vi "Plot Style Chooser Dialog.vi"(3 "Error In":errorcluster) -> (6 "Plot Style out":T1={"Plot Style"=enum."unchanged", "Histogram Type"=enum."Left Bound", "Line Tickness"=enum."unchanged", "Line Style"=enum."unchanged", "Point Style"=enum."unchanged", "Line Color"=0, "Point Color"=0, "Anti-aliased"=FALSE, "Line Color Chooser"=enum."unchanged", "Point Color Chooser"=enum."unchanged", "Line Color List"="", "Point Color List"=""}, 7 "Cancelled?":bool, 9 "Error Out":errorcluster)   [LabVIEW 2019]
uses:
  Plot Style 3.ctl
  <vilib>/measure/NI_MABase.lvlib
panel:
  in  "Cancel":bool
  in  "OK":bool
  out "Preview":waveform(dbl)(graph)
  in  "Plot Style":T1={"Plot Style"=enum."unchanged", "Histogram Type"=enum."Left Bound", "Line Tickness"=enum."unchanged", "Line Style"=enum."unchanged", "Point Style"=enum."unchanged", "Line Color"=0, "Point Color"=0, "Anti-aliased"=FALSE, "Line Color Chooser"=enum."unchanged", "Point Color Chooser"=enum."unchanged", "Line Color List"="", "Point Color List"=""}
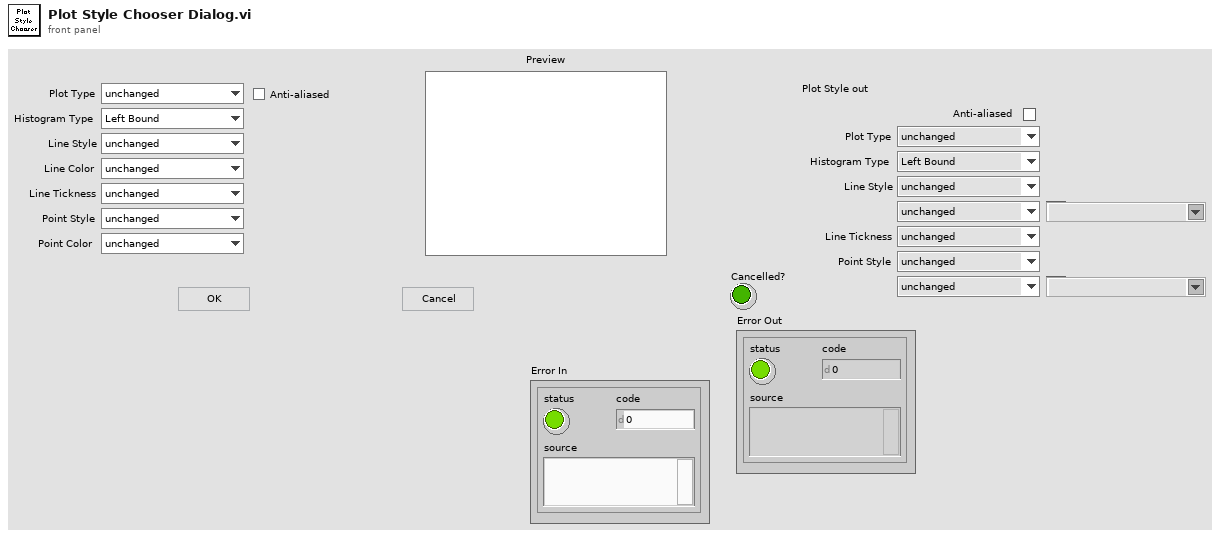
[diagram p1: front panel]
types:
  T1 = typedef "Plot Style 3.ctl" = cluster{"Plot Style":enum16{"unchanged", "Line", "Symbol", "Line + Symbol", "Histogram", "Histogram + Symbol"}, "Histogram Type":enum16{"unchanged", "Left Bound", "Center", "Right Bound"}, "Line Tickness":enum16{"unchanged", "Thin", "1 pixel", "2 pixel", "3 pixel", "4 pixel", "5 pixel"}, "Line Style":enum16{"unchanged", "Plain", "Long Dash", "Short Dash", "Long-Short Dash", "Long-Short-Short Dash"}, "Point Style":enum16{"unchanged", "None", "Empty Circle", "Filled Circle", "Thick Circle", "Dotted Circle", "Empty Square", "Filled Square", "Thick Square", "Dotted Square", "Small Filled Square", "Dot", "Cross", "Tiny Cross", "Large X", "Small x", "Diamond", "Small Empty Square"}, "Line Color":u32, "Point Color":u32, "Anti-aliased":bool, "Line Color Chooser":enum16{"unchanged", "Color Box", "Color List"}, "Point Color Chooser":enum16{"unchanged", "Color Box", "Color List"}, "Line Color List":string, "Point Color List":string}
  T2 = enum16{"Sine Wave", "Triangle Wave", "Square Wave", "Sawtooth Wave"}
  T3 = typedef "Single Plot Style 2.ctl" = cluster{"Plot Style":enum16{"unchanged", "Line", "Symbol", "Line + Symbol", "Histogram", "Histogram + Symbol"}, "Histogram Type":enum16{"unchanged", "Left Bound", "Center", "Right Bound"}, "Line Tickness":enum16{"unchanged", "Thin", "1 pixel", "2 pixel", "3 pixel", "4 pixel", "5 pixel"}, "Line Style":enum16{"unchanged", "Plain", "Long Dash", "Short Dash", "Long-Short Dash", "Long-Short-Short Dash"}, "Point Style":enum16{"unchanged", "None", "Empty Circle", "Filled Circle", "Thick Circle", "Dotted Circle", "Empty Square", "Filled Square", "Thick Square", "Dotted Square", "Small Filled Square", "Dot", "Cross", "Tiny Cross", "Large X", "Small x", "Diamond", "Small Empty Square"}, "Line Color":u32, "Line Color defined?":bool, "Point Color":u32, "Point Color defined?":bool, "Anti-aliased":bool}
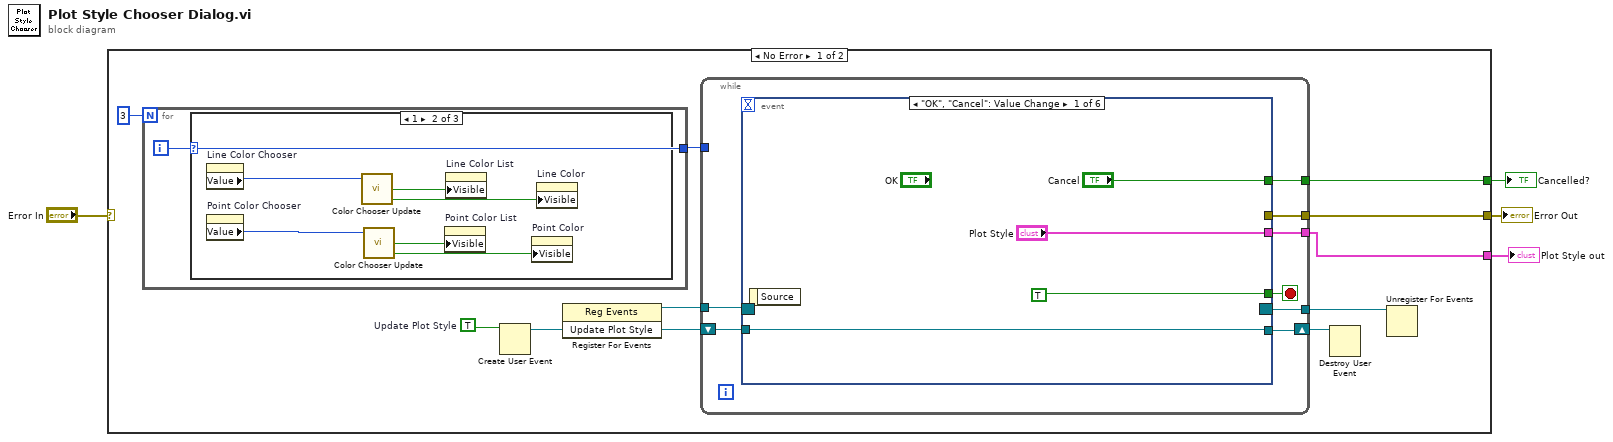
[diagram p0: block diagram]
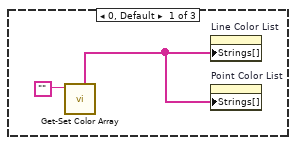
[diagram p2: hidden frame]
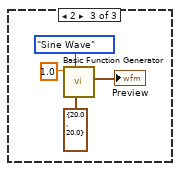
[diagram p3: hidden frame]
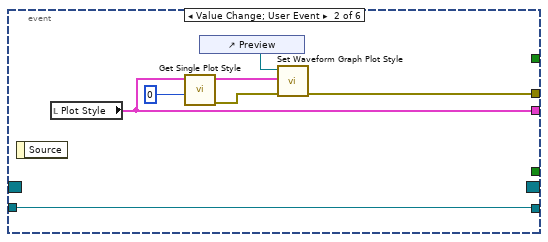
[diagram p4: hidden frame]
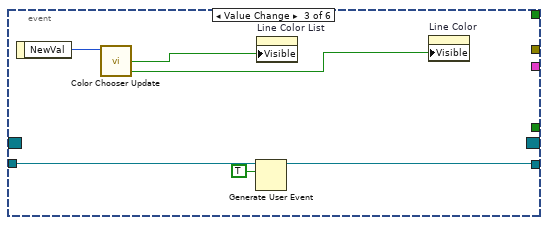
[diagram p5: hidden frame]
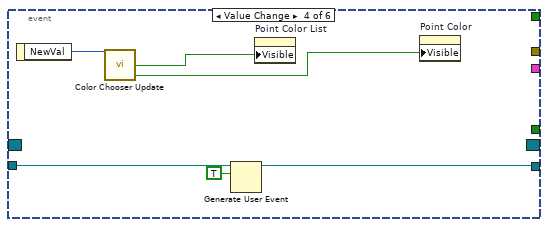
[diagram p6: hidden frame]
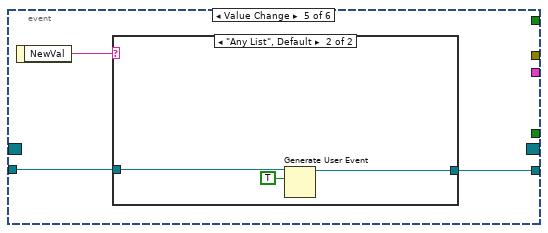
[diagram p7: hidden frame]
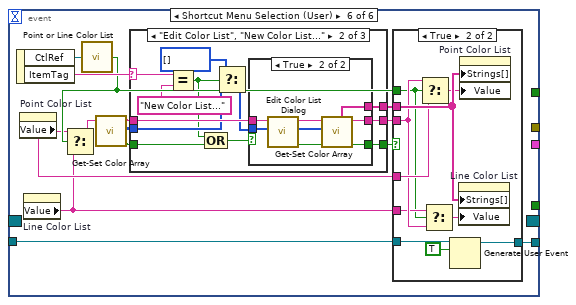
[diagram p9: hidden frame]
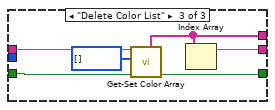
[diagram p13: hidden frame]
diagram:
  n1 = case shown="No Error" "Error In" {
    selector: "Error In" -> [_ w117]
    tunnel: [w7 w117] -> w3
    tunnel: [w6 _] -> w2
    tunnel: [w5 _] -> w1
    frame No Error {
      w12 = TRUE  # Update Plot Style
      n2 = for {
        N: 3 -> [_]
        tunnel: [w15] -> w13
        i -> [w15]
        n3 = case shown="1" w15 {
          frame 0, Default {
            n4 = call "Get-Set Color Array.vi"("Color List Name"="") -> ("Color List Name (out)"=w17:string[])  [unwired: 5 in, 5 out]
            n5 = property on="Line Color List" class="CmbBox"("Strings[]"=w17) -> ()  [unwired: 2 in, 2 out]
            n6 = property on="Point Color List" class="CmbBox"("Strings[]"=w17) -> ()  [unwired: 2 in, 2 out]
          }
          frame 1 {
            n7 = property on="Line Color Chooser" class="Enum (strict)"() -> ("Value"=w20:enum16{"unchanged", "Color Box", "Color List"})  [unwired: 2 in, 2 out]
            n8 = property on="Point Color Chooser" class="Enum (strict)"() -> ("Value"=w23:enum16{"unchanged", "Color Box", "Color List"})  [unwired: 2 in, 2 out]
            n9 = call "Color Chooser Update.vi"("Color Chooser"=w20) -> ("Color Box Visible"=w18:bool, "Color List Visible"=w19:bool)  [unwired: 3 in]
            n10 = call "Color Chooser Update.vi"("Color Chooser"=w23) -> ("Color Box Visible"=w21:bool, "Color List Visible"=w22:bool)  [unwired: 3 in]
            n11 = property on="Point Color List" class="CmbBox"("Visible"=w22) -> ()  [unwired: 2 in, 2 out]
            n12 = property on="Line Color List" class="CmbBox"("Visible"=w19) -> ()  [unwired: 2 in, 2 out]
            n13 = property on="Point Color" class="ColBox"("Visible"=w21) -> ()  [unwired: 2 in, 2 out]
            n14 = property on="Line Color" class="ColBox"("Visible"=w18) -> ()  [unwired: 2 in, 2 out]
          }
          frame 2 {
            n15 = call <vilib>:"Basic Function Generator.vi"("sampling info"=cluster{"Fs":dbl, "#s":dbl} {"Fs"=20.0, "#s"=20.0}, "signal type"=T2."Sine Wave", "frequency"=1.0) -> ("signal out"=→"Preview":waveform(dbl))  [unwired: 6 in, 2 out]
          }
        }
      }
      n16 = Create User Event(user event datatype=w12) -> (user event=w9:refnum<user-event>)  [unwired: 1 in, 1 out]
      n17 = register-events(w9) -> (reference out=w11:refnum<event-registration>)  [unwired: 2 in, 1 out]
      n18 = while {
        tunnel: [w34] -> w5
        tunnel: [w33] -> w6
        tunnel: [w32] -> w7
        tunnel: w13 -> [_]
        tunnel: w11 -> [w31]
        tunnel: [w30] -> w10
        shift-right: [w28] -> w8
        shift-left: w9 -> [w29]
        stop <- w35 stop-if-true
        n19 = event shown="[0] \"OK\", \"Cancel\": Value Change" {
          selector: w31 -> [_ _ _ _ _ _]
          dyn-events: [_ _ _ _ _ _] -> w30
          timeout: _ -> [_ _ _ _ _ _]
          tunnel: [TRUE _ _ _ _ _] -> w35
          tunnel: ["Plot Style" w40 _ _ _ _] -> w34
          tunnel: ["Cancel" _ _ _ _ _] -> w33
          tunnel: [_ w45 _ _ _ _] -> w32
          tunnel: w29 -> [w37 w41 w52 w58 w60 w73]
          tunnel: [w37 w41 w51 w57 w59 w72] -> w28
          event "OK", "Cancel": Value Change {
            n20 = event-data() -> ()  [unwired: 1 in, 1 out]
          }
          event Value Change; User Event {
            n21 = event-data() -> ()  [unwired: 1 in, 1 out]
            n22 = local read "Plot Style"() -> (w40:T1)
            n23 = call "Get Single Plot Style.vi"("index"=0, "Plot Style in"=w40) -> ("Error Out"=w42:errorcluster, "Plot Style out"=w44:T3)  [unwired: 8 in]
            n24 = control-ref of="Preview"() -> (w46:refnum<vi>)
            n25 = call "Set Waveform Graph Plot Style.vi"("Error In"=w42, "Plot Style"=w44, "Graph in"=w46) -> ("Error Out"=w45:errorcluster)  [unwired: 8 in]
          }
          event Value Change {
            n26 = event-data() -> ("NewVal"=w49:enum16{"unchanged", "Color Box", "Color List"})  [unwired: 1 in]
            n27 = call "Color Chooser Update.vi"("Color Chooser"=w49) -> ("Color Box Visible"=w47:bool, "Color List Visible"=w48:bool)  [unwired: 3 in]
            n28 = Generate User Event(user event=w52, event data cluster=TRUE ("event data")) -> (user event out=w51:refnum<user-event>)  [unwired: 2 in, 1 out]
            n29 = property on="Line Color List" class="CmbBox"("Visible"=w48) -> ()  [unwired: 2 in, 2 out]
            n30 = property on="Line Color" class="ColBox"("Visible"=w47) -> ()  [unwired: 2 in, 2 out]
          }
          event Value Change {
            n31 = event-data() -> ("NewVal"=w55:enum16{"unchanged", "Color Box", "Color List"})  [unwired: 1 in]
            n32 = call "Color Chooser Update.vi"("Color Chooser"=w55) -> ("Color Box Visible"=w53:bool, "Color List Visible"=w54:bool)  [unwired: 3 in]
            n33 = Generate User Event(user event=w58, event data cluster=TRUE ("event data")) -> (user event out=w57:refnum<user-event>)  [unwired: 2 in, 1 out]
            n34 = property on="Point Color List" class="CmbBox"("Visible"=w54) -> ()  [unwired: 2 in, 2 out]
            n35 = property on="Point Color" class="ColBox"("Visible"=w53) -> ()  [unwired: 2 in, 2 out]
          }
          event Value Change {
            n36 = event-data() -> ("NewVal"=w61:string)  [unwired: 1 in]
            n37 = case shown="\"Any List\", Default" w61 {
              tunnel: w60 -> [w62 w65]
              tunnel: [w62 w63] -> w59
              frame "" {
              }
              frame "Any List", Default {
                n38 = Generate User Event(user event=w65, event data cluster=TRUE ("event data")) -> (user event out=w63:refnum<user-event>)  [unwired: 2 in, 1 out]
              }
            }
          }
          event Shortcut Menu Selection (User) {
            n39 = event-data() -> ("CtlRef"=w71:refnum<vi>, "ItemTag"=w79:string)  [unwired: 1 in]
            n40 = property on="Point Color List" class="CmbBox"() -> ("Value"=w67:string)  [unwired: 2 in, 2 out]
            n41 = property on="Line Color List" class="CmbBox"() -> ("Value"=w66:string)  [unwired: 2 in, 2 out]
            n42 = call "Point or Line Color List.vi"("Color List"=w71) -> ("Point (T)/ Line (F)"=w69:bool)  [unwired: 8 in]
            n43 = Select(t=w67, s=w69, f=w66) -> (s? t:f=w70:string)
            n44 = call "Get-Set Color Array.vi"("Color List Name"=w70) -> ("Found?"=w76:bool, "Color Array (out)"=w77:u32[], "Color List Name (dup)"=w78:string)  [unwired: 5 in, 3 out]
            n45 = case shown="\"Edit Color List\", \"New Color List...\"" w79 {
              selector: w79 -> [_ w99 _]
              tunnel: w78 -> [_ w97 w116]
              tunnel: w77 -> [_ w96 _]
              tunnel: w76 -> [_ w102 w114]
              tunnel: [_ w101 w113] -> w75
              tunnel: [_ w100 w112] -> w74
              tunnel: [_ w91 w111] -> w68
              frame "", Default {
              }
              frame "Edit Color List", "New Color List..." {
                n46 = Equal?(x=w99, y="New Color List...") -> (x = y?=w92:bool)
                n47 = Compound Arithmetic op=OR(w92, w102) -> (w93:bool)
                n48 = Select(t=u32[] [], s=w92, f=w96) -> (s? t:f=w94:u32[])
                n49 = case shown="True" w93 {
                  tunnel: w97 -> [_ w110]
                  tunnel: w94 -> [_ w109]
                  tunnel: [_ w105] -> w101
                  tunnel: [_ w104] -> w100
                  tunnel: [_ w103] -> w91
                  frame False {
                  }
                  frame True {
                    n50 = call "Edit Color List Dialog.vi"("Color List"=w109, "Color List Name"=w110) -> ("OK?"=w106:bool, "Color List (out)"=w107:u32[], "Color List Name (out)"=w108:string)  [unwired: 7 in]
                    n51 = call "Get-Set Color Array.vi"("Get (F)/Set (T)"=w106, "Color Array (in)"=w107, "Color List Name"=w108) -> ("Found?"=w105:bool, "Color List Name (dup)"=w103:string, "Color List Name (out)"=w104:string[])  [unwired: 3 in, 3 out]
                  }
                }
              }
              frame "Delete Color List" {
                n52 = call "Get-Set Color Array.vi"("Get (F)/Set (T)"=w114, "Color Array (in)"=u32[] [], "Color List Name"=w116) -> ("Found?"=w113:bool, "Color List Name (out)"=w112:string[])  [unwired: 3 in, 4 out]
                n53 = Index Array(array=w112) -> (element=w111:string)  [unwired: 1 in]
              }
            }
            n54 = case shown="True" w75 {
              tunnel: w74 -> [_ w90]
              tunnel: w73 -> [w80 w89]
              tunnel: [w80 w88] -> w72
              tunnel: w69 -> [_ w81]
              tunnel: w68 -> [_ w83]
              tunnel: w67 -> [_ w85]
              tunnel: w66 -> [_ w82]
              frame False {
              }
              frame True {
                n55 = Select(t=w83, s=w81, f=w85) -> (s? t:f=w86:string)
                n56 = Select(t=w82, s=w81, f=w83) -> (s? t:f=w84:string)
                n57 = Generate User Event(user event=w89, event data cluster=TRUE ("event data")) -> (user event out=w88:refnum<user-event>)  [unwired: 2 in, 1 out]
                n58 = property on="Line Color List" class="CmbBox"("Strings[]"=w90, "Value"=w84) -> ()  [unwired: 2 in, 2 out]
                n59 = property on="Point Color List" class="CmbBox"("Strings[]"=w90, "Value"=w86) -> ()  [unwired: 2 in, 2 out]
              }
            }
          }
        }
      }
      n60 = Destroy User Event(user event=w8) -> ()  [unwired: 1 in, 1 out]
      n61 = Unregister For Events(event registration refnum=w10) -> ()  [unwired: 1 in, 1 out]
    }
    frame Error {
    }
  }
  "Error Out" <- w3
  "Cancelled?" <- w2
  "Plot Style out" <- w1
